vi "SearchClsterArrInd.vi"(8 "ErrorIn(No Error)":errorcluster caption="entrée d'erreur (pas d'erreur)", 9 "ScanlistSize":i32=-1, 10 "array":cluster{"Tableau":i32[]}[](array[cluster]), 11 "Currtaskparcnt":i32) -> (0 "sortie d'erreur":errorcluster, 2 "output array":cluster{"Tableau":i32[]}[](array[cluster]))   [LabVIEW 2019]
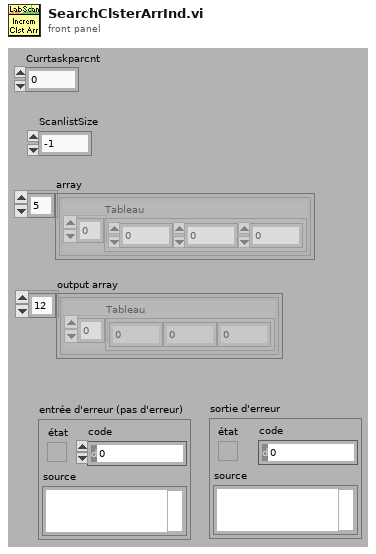
[diagram p1: front panel]
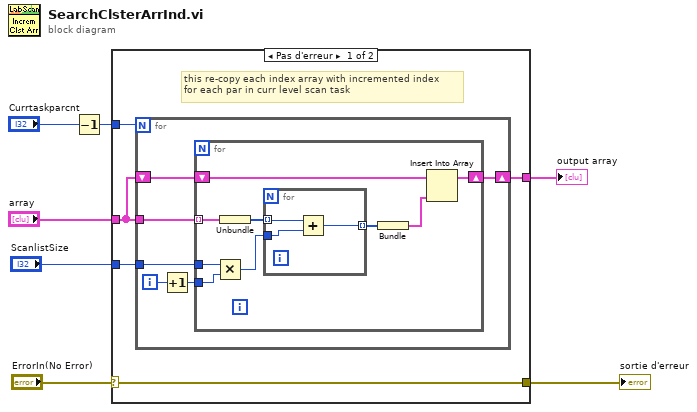
[diagram p0: block diagram]
diagram:
  n1 = Decrement(x="Currtaskparcnt") -> (x-1=w1:i32)
  n2 = case shown="Pas d'erreur" "ErrorIn(No Error)" {
    selector: "ErrorIn(No Error)" -> [w11 w32]
    tunnel: [w11 w32] -> w6
    tunnel: "ScanlistSize" -> [w12 _]
    tunnel: "array" -> [w9 w31]
    tunnel: [w10 w31] -> w4
    tunnel: w1 -> [w8 _]
    frame No Error {
      # "this re-copy each index array with incremented index\nfor each par in curr level scan task"
      n3 = for {
        N: w8 -> [_]
        tunnel: w12 -> [w18]
        shift-right: [w16] -> w10
        shift-left: w9 -> [w17]
        tunnel: w9 -> [w15]
        i -> [w14]
        n4 = Increment(x=w14) -> (x+1=w13:i32)
        n5 = for {
          tunnel: w18 -> [w26]
          tunnel: w15 -> [w22] mode=indexing
          shift-right: [w23] -> w16
          shift-left: w17 -> [w21]
          tunnel: w13 -> [w19]
          n6 = Multiply(x=w26, y=w19) -> (x*y=w20:i32)
          n7 = Unbundle(w22) -> ("Tableau"=w27:i32[])
          n8 = for {
            tunnel: w27 -> [w29] mode=indexing
            tunnel: w20 -> [w30]
            tunnel: [w28] -> w25 mode=indexing
            n9 = Add(x=w29, y=w30) -> (x+y=w28:i32)
          }
          n10 = Bundle(w25) -> (w24:cluster{i32[]})  [unwired: 1 in]
          n11 = Insert Into Array(array=w21, new element=w24) -> (w23:cluster{"Tableau":i32[]}[])  [unwired: 1 in]
        }
      }
    }
    frame Error {
    }
  }
  "sortie d'erreur" <- w6
  "output array" <- w4
